vi "start.vi"(8 "error in (no error)":errorcluster, 10 "AcqConfig":T1 {"TC 2 Offset" format="%#_f"; "TC 2 Scale" format="%#_f"; "TC 1 Offset" format="%#_f"; "TC 1 Scale" format="%#_f"}, 11 "Handle In":i32) -> (0 "error out":errorcluster, 3 "Handle Out":i32)   [LabVIEW 2025, in "LabJackEKG.lvlib"]
uses:
  LabJackEKG.lvlib
  Typedefs/AcqusitionConfig.ctl
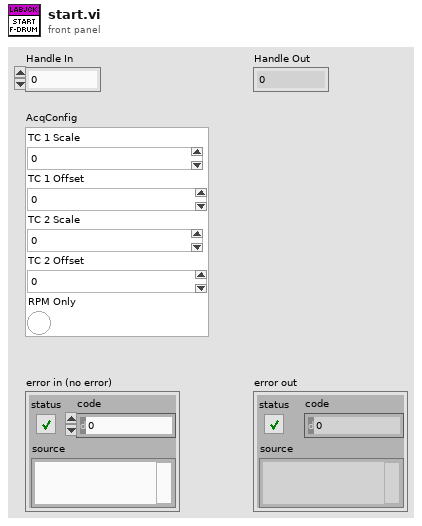
[diagram p1: front panel]
types:
  T1 = typedef "LabJackEKG.lvlib/AcqusitionConfig.ctl" = cluster{"TC 1 Scale":dbl, "TC 1 Offset":dbl, "TC 2 Scale":dbl, "TC 2 Offset":dbl, "RPM Only":bool}
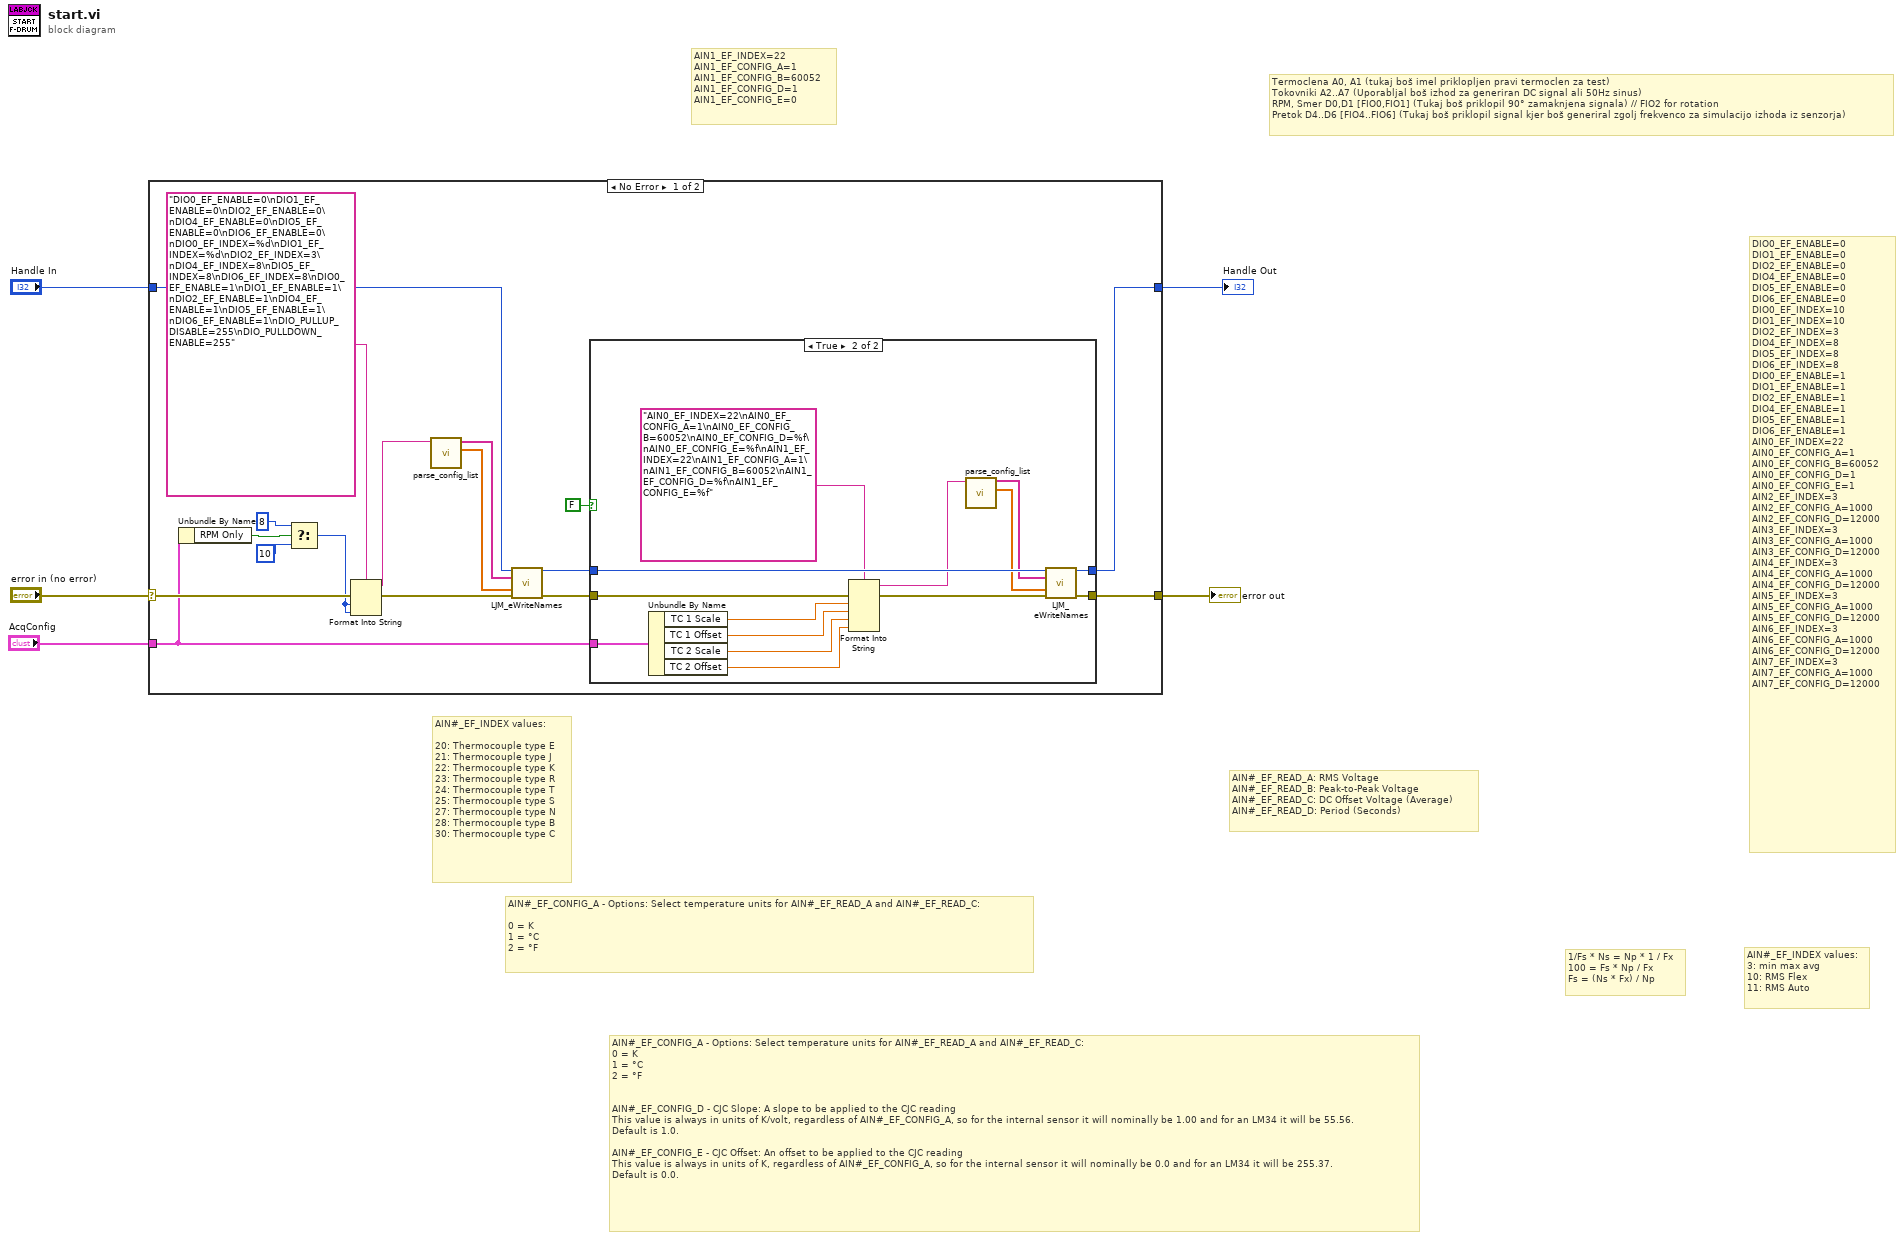
[diagram p0: block diagram]
diagram:
  # "DIO0_EF_ENABLE=0\nDIO1_EF_ENABLE=0\nDIO2_EF_ENABLE=0\nDIO4_EF_ENABLE=0\nDIO5_EF_ENABLE=0\nDIO6_EF_ENABLE=0\nDIO0_EF_INDEX=10\nDIO1_EF_INDEX=10\nDIO2_EF_INDEX=3\nDIO4_EF_INDEX=8\nDIO5_EF_INDEX=8\nDIO6_EF_INDEX=8\nDIO0_EF_ENABLE=1\nDIO1_EF_ENABLE=1\nDIO2_EF_ENABLE=1\nDIO4_EF_ENABLE=1\nDIO5_EF_ENABLE=1\nDIO6_EF_ENABLE=1\nAIN0_EF_INDEX=22\nAIN0_EF_CONFIG_A=1\nAIN0_EF_CONFIG_B=60052\nAIN0_EF_CONFIG_D=1\nAIN0_EF_CONFIG_E=1\nAIN2_EF_INDEX=3\nAIN2_EF_CONFIG_A=1000\nAIN2_EF_CONFIG_D=12000\nAIN3_EF_INDEX=3\nAIN3_EF_CONFIG_A=1000\nAIN3_EF_CONFIG_D=12000\nAIN4_EF_INDEX=3\nAIN4_EF_CONFIG_A=1000\nAIN4_EF_CONFIG_D=12000\nAIN5_EF_INDEX=3\nAIN5_EF_CONFIG_A=1000\nAIN5_EF_CONFIG_D=12000\nAIN6_EF_INDEX=3\nAIN6_EF_CONFIG_A=1000\nAIN6_EF_CONFIG_D=12000\nAIN7_EF_INDEX=3\nAIN7_EF_CONFIG_A=1000\nAIN7_EF_CONFIG_D=12000"
  # "1/Fs * Ns = Np * 1 / Fx\n100 = Fs * Np / Fx\nFs = (Ns * Fx) / Np"
  # "AIN1_EF_INDEX=22\nAIN1_EF_CONFIG_A=1\nAIN1_EF_CONFIG_B=60052\nAIN1_EF_CONFIG_D=1\nAIN1_EF_CONFIG_E=0"
  # "AIN#_EF_INDEX values:\n3: min max avg\n10: RMS Flex\n11: RMS Auto"
  # "AIN#_EF_READ_A: RMS Voltage\nAIN#_EF_READ_B: Peak-to-Peak Voltage\nAIN#_EF_READ_C: DC Offset Voltage (Average)\nAIN#_EF_READ_D: Period (Seconds)"
  # "AIN#_EF_CONFIG_A - Options: Select temperature units for AIN#_EF_READ_A and AIN#_EF_READ_C:\n0 = K\n1 = °C\n2 = °F\n\n\nAIN#_EF_CONFIG_D - CJC Slope: A slope to be applied to the CJC reading\nThis value is always in units of K/volt, regardless of AIN#_EF_CONFIG_A, so for the internal sensor it will nominally be 1.00 and for an LM34 it will be 55.56.\nDefault is 1.0.\n\nAIN#_EF_CONFIG_E - CJC Offset: An offset to be applied to the CJC reading\nThis value is always in units of K, regardless of AIN#_EF_CONFIG_A, so for the internal sensor it will nominally be 0.0 and for an LM34 it will be 255.37.\nDefault is 0.0."
  # "AIN#_EF_CONFIG_A - Options: Select temperature units for AIN#_EF_READ_A and AIN#_EF_READ_C:\n\n0 = K\n1 = °C\n2 = °F"
  # "AIN#_EF_INDEX values:\n\n20: Thermocouple type E\n21: Thermocouple type J\n22: Thermocouple type K\n23: Thermocouple type R\n24: Thermocouple type T \n25: Thermocouple type S\n27: Thermocouple type N\n28: Thermocouple type B\n30: Thermocouple type C"
  # "Termoclena A0, A1 (tukaj boš imel priklopljen pravi termoclen za test)\nTokovniki A2..A7 (Uporabljal boš izhod za generiran DC signal ali 50Hz sinus)\nRPM, Smer D0,D1 [FIO0,FIO1] (Tukaj boš priklopil 90° zamaknjena signala) // FIO2 for rotation\nPretok D4..D6 [FIO4..FIO6] (Tukaj boš priklopil signal kjer boš generiral zgolj frekvenco za simulacijo izhoda iz senzorja)"
  n1 = case shown="No Error" "error in (no error)" {
    selector: "error in (no error)" -> [w22 w40]
    tunnel: [w17 w39] -> w5
    tunnel: "Handle In" -> [w21 w39]
    tunnel: [w16 w40] -> w2
    tunnel: "AcqConfig" -> [w7 _]
    frame No Error {
      n2 = Unbundle By Name(w7) -> ("RPM Only"=w6:bool)
      n3 = Select(t=8, s=w6, f=10) -> (s? t:f=w8:i32)
      n4 = Format Into String(format string="DIO0_EF_ENABLE=0\nDIO1_EF_ENABLE=0\nDIO2_EF_ENABLE=0\nDIO4_EF_ENABLE=0\nDIO5_EF_ENABLE=0\nDIO6_EF_ENABLE=0\nDIO0_EF_INDEX=%d\nDIO1_EF_INDEX=%d\nDIO2_EF_INDEX=3\nDIO4_EF_INDEX=8\nDIO5_EF_INDEX=8\nDIO6_EF_INDEX=8\nDIO0_EF_ENABLE=1\nDIO1_EF_ENABLE=1\nDIO2_EF_ENABLE=1\nDIO4_EF_ENABLE=1\nDIO5_EF_ENABLE=1\nDIO6_EF_ENABLE=1\nDIO_PULLUP_DISABLE=255\nDIO_PULLDOWN_ENABLE=255", error in=w22, w8, w8) -> (resulting string=w11:string, error out=w13:errorcluster)  [unwired: 1 in]
      n5 = call "parse_config_list.vi"("String"=w11) -> ("Values"=w20:dbl[], "Names"=w19:string[])  [unwired: 9 in]
      n6 = call <vilib>:"LJM_eWriteNames.vi"("Handle In"=w21, "aNames"=w19, "aValuesIn"=w20, "error in"=w13) -> ("Handle Out"=w18:i32, "error out"=w15:errorcluster)  [unwired: 9 in, 1 out]
      n7 = case shown="True" FALSE {
        tunnel: w18 -> [w24 w38]
        tunnel: [w24 w35] -> w17
        tunnel: [w23 w34] -> w16
        tunnel: w15 -> [w23 w31]
        tunnel: w7 -> [_ w29]
        frame False {
        }
        frame True {
          n8 = Unbundle By Name(w29) -> ("TC 1 Scale"=w28:dbl, "TC 1 Offset"=w27:dbl, "TC 2 Scale"=w26:dbl, "TC 2 Offset"=w25:dbl)
          n9 = Format Into String(format string="AIN0_EF_INDEX=22\nAIN0_EF_CONFIG_A=1\nAIN0_EF_CONFIG_B=60052\nAIN0_EF_CONFIG_D=%f\nAIN0_EF_CONFIG_E=%f\nAIN1_EF_INDEX=22\nAIN1_EF_CONFIG_A=1\nAIN1_EF_CONFIG_B=60052\nAIN1_EF_CONFIG_D=%f\nAIN1_EF_CONFIG_E=%f", error in=w31, w28, w27, w26, w25) -> (resulting string=w33:string, error out=w30:errorcluster)  [unwired: 1 in]
          n10 = call "parse_config_list.vi"("String"=w33) -> ("Values"=w37:dbl[], "Names"=w36:string[])  [unwired: 9 in]
          n11 = call <vilib>:"LJM_eWriteNames.vi"("Handle In"=w38, "aNames"=w36, "aValuesIn"=w37, "error in"=w30) -> ("Handle Out"=w35:i32, "error out"=w34:errorcluster)  [unwired: 9 in, 1 out]
        }
      }
    }
    frame Error {
    }
  }
  "error out" <- w2
  "Handle Out" <- w5
